vi "Sudoku Calculation New.vi"(8 "error in (no error)":errorcluster, 11 "Sudoku Class in":refnum<class "Sudoku Class.lvclass">) -> (0 "error out":errorcluster, 3 "Sudoku Class out":refnum<class "Sudoku Class.lvclass">)   [LabVIEW 2015, in "Sudoku Library.lvlib" / "Sudoku Class.lvclass"]
doc: "Created IvanLis by LabVIEW Portal\nProfile: http://labviewportal.org/memberlist.php?mode=viewprofile&u=987\neMail: IvanLisanov@gMail.com\nTelegram: https://t.me/IvanLis"
uses:
  Sudoku Class.lvclass
  TypeDef/Sudoku Formal.ctl
  TypeDef/Cell Formal.ctl
  TypeDef/Calculation State.ctl
  Sudoku Class.lvclass/Sudoku Class.ctl
  Sudoku Library.lvlib
panel:
  out "Calculation State 2":T1
  out "Calculation State":T1
  out "Formal Size":i32[][](array[numeric])
  out "Sudoku Formal In":T2
  out "Sudoku Int In":u8[][](array[numeric])
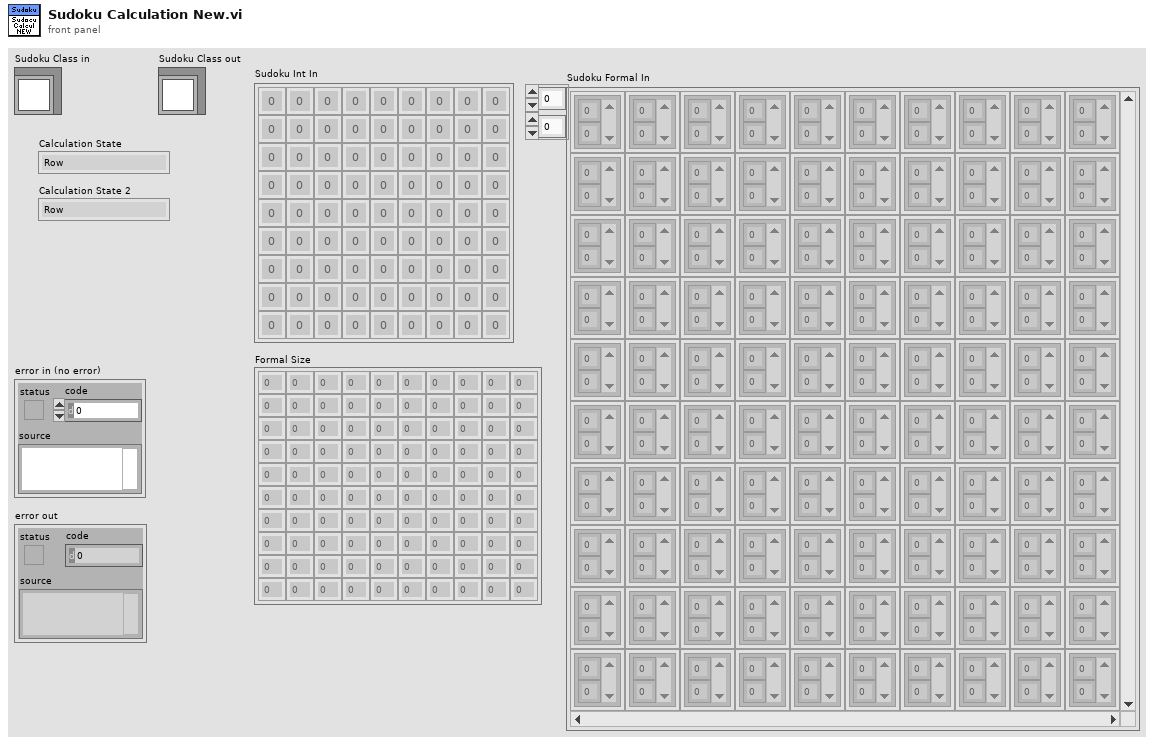
[diagram p1: front panel]
types:
  T1 = typedef "Sudoku Library.lvlib/Calculation State.ctl" = enum16{"Row", "Column", "Square"}
  T2 = typedef "Sudoku Library.lvlib/Sudoku Formal.ctl" = T3[][]
  T3 = typedef "Sudoku Library.lvlib/Cell Formal.ctl" = cluster{"Variant":u8[]}
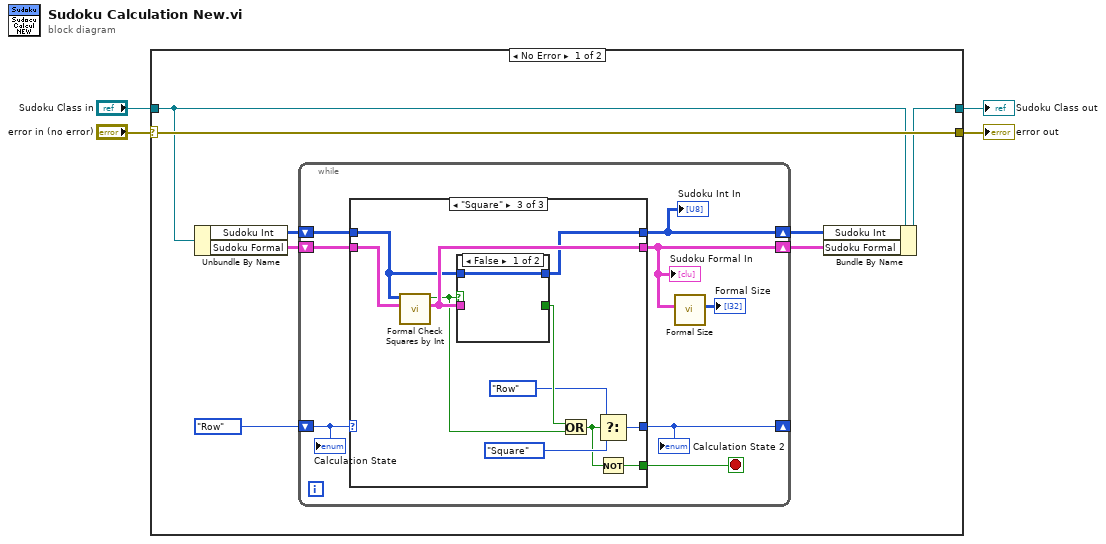
[diagram p0: block diagram]
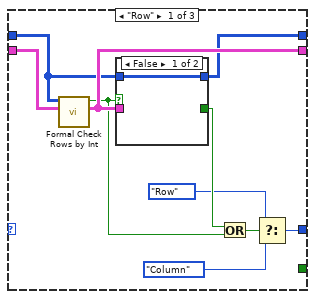
[diagram p2: hidden frame]
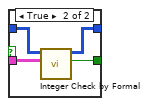
[diagram p3: hidden frame]
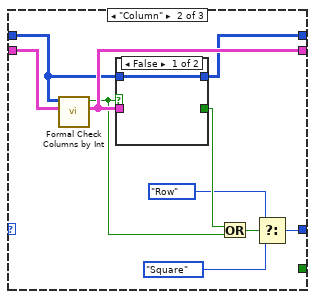
[diagram p4: hidden frame]
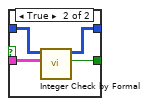
[diagram p5: hidden frame]
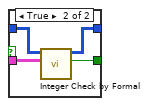
[diagram p6: hidden frame]
diagram:
  n1 = case shown="No Error" "error in (no error)" {
    selector: "error in (no error)" -> [w12 w68]
    tunnel: [w12 w68] -> w3
    tunnel: [w8 w67] -> w1
    tunnel: "Sudoku Class in" -> [w11 w67]
    frame No Error {
      n2 = Unbundle By Name(w11) -> ("Sudoku Int"=w10:u8[][], "Sudoku Formal"=w9:T2)
      n3 = while {
        shift-right: [w15] -> w7
        shift-left: w10 -> [w20]
        shift-right: [w14] -> w6
        shift-left: w9 -> [w19]
        shift-right: [w17] -> _
        shift-left: Calculation_State."Row" -> [w18]
        stop <- w16 stop-if-true
        n4 = case shown="\"Square\"" w18 {
          tunnel: w20 -> [w27 w42 w58]
          tunnel: w19 -> [w30 w45 w61]
          tunnel: [w26 w41 w57] -> w15
          tunnel: [w28 w43 w59] -> w14
          tunnel: [w29 w44 w60] -> w17
          tunnel: [_ _ w51] -> w16
          frame "Row" {
            n5 = call "Formal Check Rows by Int.vi"("Sudoku Formal In"=w30, "Sudoku Int"=w27) -> ("Sudoku Formal Out"=w28:T2, "Is Modify"=w23:bool)  [unwired: 8 in]
            n6 = case shown="False" w23 {
              tunnel: w28 -> [_ w35]
              tunnel: w27 -> [w31 w34]
              tunnel: [w31 w33] -> w26
              tunnel: [_ w32] -> w24
              frame False {
              }
              frame True {
                n7 = call "Integer Check by Formal.vi"("Sudoku Formal In"=w35, "Sudoku Int In"=w34) -> ("Is Modify"=w32:bool, "Sudoku Int Out"=w33:u8[][])  [unwired: 8 in]
              }
            }
            n8 = Or(x=w24, y=w23) -> (x .or. y?=w25:bool)
            n9 = Select(t=Calculation_State."Row", s=w25, f=Calculation_State."Column") -> (s? t:f=w29:T1)
          }
          frame "Column" {
            n10 = call "Formal Check Columns by Int.vi"("Sudoku Formal In"=w45, "Sudoku Int"=w42) -> ("Sudoku Formal Out"=w43:T2, "Is Modify"=w38:bool)  [unwired: 8 in]
            n11 = case shown="False" w38 {
              tunnel: w43 -> [_ w50]
              tunnel: w42 -> [w46 w49]
              tunnel: [w46 w48] -> w41
              tunnel: [_ w47] -> w39
              frame False {
              }
              frame True {
                n12 = call "Integer Check by Formal.vi"("Sudoku Formal In"=w50, "Sudoku Int In"=w49) -> ("Is Modify"=w47:bool, "Sudoku Int Out"=w48:u8[][])  [unwired: 8 in]
              }
            }
            n13 = Or(x=w39, y=w38) -> (x .or. y?=w40:bool)
            n14 = Select(t=Calculation_State."Row", s=w40, f=Calculation_State."Square") -> (s? t:f=w44:T1)
          }
          frame "Square" {
            n15 = call "Formal Check Squares by Int.vi"("Sudoku Formal In"=w61, "Sudoku Int"=w58) -> ("Sudoku Formal Out"=w59:T2, "Is Modify"=w55:bool)  [unwired: 8 in]
            n16 = case shown="False" w55 {
              tunnel: w59 -> [_ w66]
              tunnel: w58 -> [w62 w65]
              tunnel: [w62 w64] -> w57
              tunnel: [_ w63] -> w56
              frame False {
              }
              frame True {
                n17 = call "Integer Check by Formal.vi"("Sudoku Formal In"=w66, "Sudoku Int In"=w65) -> ("Is Modify"=w63:bool, "Sudoku Int Out"=w64:u8[][])  [unwired: 8 in]
              }
            }
            n18 = Or(x=w56, y=w55) -> (x .or. y?=w52:bool)
            n19 = Select(t=Calculation_State."Row", s=w52, f=Calculation_State."Square") -> (s? t:f=w60:T1)
            n20 = Not(x=w52) -> (.not. x?=w51:bool)
          }
        }
        "Sudoku Int In" <- w15
        "Sudoku Formal In" <- w14
        "Calculation State 2" <- w17
        n21 = call "Formal Size.vi"("Sudoku Formal In"=w14) -> ("Formal Size"=→"Formal Size":i32[][])  [unwired: 10 in]
        "Calculation State" <- w18
      }
      n22 = Bundle By Name(cluster=w11, "Sudoku Int"=w7, "Sudoku Formal"=w6) -> (w8:refnum<class "Sudoku Class.lvclass">)
    }
    frame Error {
    }
  }
  "error out" <- w3
  "Sudoku Class out" <- w1
